vi "UHR-Fleezers Control (host) -Leonardo 04-2018 V2_sym.vi"(0 "Tab Control":T5(tab)=enum."Trap Control (RF)") -> ()   [LabVIEW 2013] (continued)
                      n1852 = Delete From Array(array=w3581, index=0) -> (array with subset deleted=w3579:cluster{"f0":dbl, "df":dbl, "magnitude":dbl[]}[])  [unwired: 1 in, 1 out]
                    }
                  }
                }
                frame True {
                  n1853 = Build Array(w3583) -> (w3582:cluster{"f0":dbl, "df":dbl, "magnitude":dbl[]}[])
                }
              }
              n1854 = for {
                tunnel: w3553 -> [w3572] mode=indexing
                tunnel: [w3571] -> w3563 mode=indexing
                workers-P: _ -> [_]
                n1855 = Unbundle By Name(w3572) -> ("magnitude"=w3571:dbl[])
              }
              n1856 = Transpose 2D Array(2D array=w3563) -> (transposed array=w3562:dbl[][])
              n1857 = for {
                tunnel: w3562 -> [w3570] mode=indexing
                tunnel: [w3569] -> w3561 mode=indexing
                workers-P: _ -> [_]
                n1858 = Add Array Elements(numeric array=w3570) -> (sum=w3569:dbl)
              }
              n1859 = Select(t=w3556, s=w3557, f=w3555) -> (s? t:f=w3554:dbl)
              n1860 = Divide(x=w3561, y=w3554) -> (x/y=w3559:dbl[])
              n1861 = Bundle By Name(cluster=w3560, "magnitude"=w3559) -> (w3558:cluster{"f0":dbl, "df":dbl, "magnitude":dbl[]})
            }
          }
        }
        n1862 = case shown="True" w3500 {
          tunnel: w3501 -> [w3532 w3538]
          tunnel: [w3532 w3533] -> w3499
          frame False {
          }
          frame True {
            n1863 = Array Subset(array=w3538, index (row)=0 ("index"), length (row)=4 ("length"), index (col)=0 ("index"), length (col)=1 ("length")) -> (w3533:T47)
          }
        }
        n1864 = feedback-in #9(w3499) -> ()
        n1865 = Split 1D Array(array=w3513, index=2) -> (first subarray=→"FFT 1":cluster{"f0":dbl, "df":dbl, "magnitude":dbl[]}[], second subarray=→"FFT 2":cluster{"f0":dbl, "df":dbl, "magnitude":dbl[]}[])
      }
    }
    n1866 = Index Array(array=w2395, index=1) -> (element=w2403:waveform(dbl))
    n1867 = case "For displaying the high resolution display (no downsampling)" shown="True" w2459 {
      tunnel: w2422 -> [_ w2741]
      frame False {
      }
      frame True {
        n1868 = Index Array(array=w2741, index="High Res. Display") -> (element=w2742:waveform(dbl))
        n1869 = call <vilib>:"Std Deviation and Variance.vi"("X"=w2742) -> ("mean"=w2749:dbl, "standard deviation"=w2754:dbl)  [unwired: 1 in, 1 out]
        "Mean Intensity" <- w2749
        "Sigma" <- w2754
        n1870 = Subtract(x=w2742, y=w2749) -> (x-y=w2748:waveform(dbl))
        n1871 = Select(t=w2748, s="Subtract mean", f=w2742) -> (s? t:f=→"1 Channel":waveform(dbl))
        n1872 = Divide(x=w2754, y=w2749) -> (x/y=→"Sigma/Mean":dbl)
        n1873 = feedback #10(1) -> (w2743:i32)
        n1874 = Greater Or Equal?(x=w2743, y="Slow mean N ave.") -> (x >= y?=w2756:bool)
        n1875 = Increment(x=w2743) -> (x+1=w2758:i32)
        n1876 = Select(t=1, s=w2756, f=w2758) -> (s? t:f=w2745:i32)
        n1877 = feedback-in #10(w2745) -> ()
        n1878 = feedback #11() -> (w2746:waveform(dbl))  [unwired: 1 out]
        n1879 = case shown="Default" w2743 {
          tunnel: [w2761 w2764] -> w2747
          tunnel: w2746 -> [w2763 _]
          tunnel: w2742 -> [w2762 w2764]
          frame Default {
            n1880 = call-poly <vilib>:"Append Waveforms.vi"("waveform B"=w2762, "waveform A"=w2763) -> ("waveform out"=w2761:waveform(dbl))  [unwired: 1 in, 8 out]
          }
          frame 1 {
          }
        }
        n1881 = feedback-in #11(w2747) -> ()
        n1882 = case shown="True" w2756 {
          tunnel: w2747 -> [_ w2760]
          frame False {
          }
          frame True {
            n1883 = call-poly <vilib>:"Mean.vi"("X"=w2760) -> ("mean"=→"Slow mean":dbl)  [unwired: 1 out]
          }
        }
      }
    }
    n1884 = case "For plotting results of scanning MCL" shown="True" w2529 {
      tunnel: w2528 -> [_ w2881]
      tunnel: w2452 -> [_ w2977]
      tunnel: w2537 -> [_ _]
      tunnel: w2422 -> [_ w2951]
      tunnel: w2397 -> [_ w2882]
      tunnel: w2396 -> [_ w2855]
      frame False {
      }
      frame True {
        w2862 = u32 0 items=["Horizontal", "Vertical", "Central", "1st Diagonal", "2nd Diagonal"] ("Type of Symmetry")
        w2890 = u32 0 items=["Horizontal", "Vertical", "Central", "1st Diagonal", "2nd Diagonal"] ("Type of Symmetry")
        w2893 = u32 0 items=["Horizontal", "Vertical", "Central", "1st Diagonal", "2nd Diagonal"] ("Type of Symmetry")
        w2922 = u32 0 items=["Horizontal", "Vertical", "Central", "1st Diagonal", "2nd Diagonal"] ("Type of Symmetry")
        n1885 = Index Array(array=w2951, index=10) -> (element=w2957:waveform(dbl))
        n1886 = Index Array(array=w2951, index=11) -> (element=w2954:waveform(dbl))
        n1887 = local read "Cycles/step (MCL)"() -> (w2907:u64)
        n1888 = Index Array(array=w2951, index="Channel") -> (element=w2953:waveform(dbl))
        n1889 = Unbundle(w2855) -> ("New Image"=w2854:T3, "New Image"=w2853:T3, "New Image"=w2852:T3, "New Image"=w2851:T3)
        n1890 = Unbundle By Name(w2957) -> ("Y"=w2909:dbl[])
        n1891 = Unbundle By Name(w2954) -> ("Y"=w2911:dbl[])
        n1892 = Unbundle By Name(w2953) -> ("Y"=w2916:dbl[])
        n1893 = call "downsample 1D array - double.vi"("Ave N"=w2907, "Array In"=w2909) -> ("Array Out"=w2908:dbl[])  [unwired: 1 out]
        n1894 = call "downsample 1D array - double.vi"("Ave N"=w2907, "Array In"=w2911) -> ("Array Out"=w2910:dbl[])  [unwired: 1 out]
        n1895 = call "downsample 1D array - double.vi"("Ave N"=w2907, "Array In"=w2916) -> ("Array Out"=w2915:dbl[])  [unwired: 1 out]
        n1896 = feedback #12(w2977) -> (w2978:dbl[])
        n1897 = Build Array (concatenate)(w2978, w2977) -> (w2959:dbl[])
        n1898 = feedback #13(w2882) -> (w2884:dbl[])
        n1899 = Build Array (concatenate)(w2884, w2882) -> (w2883:dbl[])
        n1900 = local read "Scan steps (MCL)"() -> (w2864:u64)
        n1901 = Select(t=w2977, s=w2881, f=w2959) -> (s? t:f=w2963:dbl[])
        n1902 = feedback-in #12(w2963) -> ()
        n1903 = Select(t=w2882, s=w2881, f=w2883) -> (s? t:f=w2865:dbl[])
        n1904 = feedback-in #13(w2865) -> ()
        n1905 = local read "Scan lines (y)"() -> (w2850:u64)
        n1906 = local read "N APD Samp/step"() -> (w2866:dbl)
        n1907 = feedback #14(w2908) -> (w2965:dbl[])
        n1908 = Build Array (concatenate)(w2965, w2908) -> (w2956:dbl[])
        n1909 = feedback #15(w2915) -> (w2975:dbl[])
        n1910 = Build Array (concatenate)(w2975, w2915) -> (w2974:dbl[])
        n1911 = feedback #16(w2910) -> (w2967:dbl[])
        n1912 = Build Array (concatenate)(w2967, w2910) -> (w2968:dbl[])
        n1913 = Select(t=w2908, s=w2881, f=w2956) -> (s? t:f=w2912:dbl[])
        n1914 = feedback-in #14(w2912) -> ()
        n1915 = Select(t=w2915, s=w2881, f=w2974) -> (s? t:f=w2914:dbl[])
        n1916 = feedback-in #15(w2914) -> ()
        n1917 = Select(t=w2910, s=w2881, f=w2968) -> (s? t:f=w2913:dbl[])
        n1918 = feedback-in #16(w2913) -> ()
        n1919 = Multiply(x=w2864, y=u64 2) -> (x*y=w2849:u64)
        n1920 = call "integrate 1D array interval - double.vi"("Ave N"=w2866, "Array In"=w2865) -> ("Array Out"=w2877:dbl[])  [unwired: 1 out]
        n1921 = call "integrate 1D array interval - double.vi"("Ave N"=w2866, "Array In"=w2963) -> ("Array Out"=w2962:dbl[])  [unwired: 1 out]
        n1922 = Array Size(array=w2877) -> (size(s)=w2878:i32)
        n1923 = Array Size(array=w2962) -> (size(s)=w2964:i32)
        n1924 = Multiply(x=w2850, y=w2849) -> (x*y=w2880:u64)
        n1925 = Multiply(x=w2850, y=w2849) -> (x*y=w2972:u64)
        n1926 = call-poly <vilib>:"Mean.vi"("X"=w2912) -> ("mean"=w2896:dbl)  [unwired: 1 out]
        n1927 = Subtract(x=w2880, y=w2878) -> (x-y=w2871:u64)
        n1928 = call-poly <vilib>:"Mean.vi"("X"=w2914) -> ("mean"=w2901:dbl)  [unwired: 1 out]
        n1929 = call-poly <vilib>:"Mean.vi"("X"=w2913) -> ("mean"=w2899:dbl)  [unwired: 1 out]
        n1930 = call-poly <vilib>:"Mean.vi"("X"=w2877) -> ("mean"=w2868:dbl)  [unwired: 1 out]
        n1931 = Subtract(x=w2972, y=w2964) -> (x-y=w2906:u64)
        n1932 = call-poly <vilib>:"Mean.vi"("X"=w2962) -> ("mean"=w2903:dbl)  [unwired: 1 out]
        n1933 = Initialize Array(1.0 ("element"), w2871) -> (w2867:dbl[])
        n1934 = Initialize Array(1.0 ("element"), w2906) -> (w2897:dbl[])
        n1935 = Multiply(x=w2867, y=w2868) -> (x*y=w2869:dbl[])
        n1936 = Multiply(x=w2897, y=w2899) -> (x*y=w2900:dbl[])
        n1937 = Multiply(x=w2897, y=w2901) -> (x*y=w2902:dbl[])
        n1938 = Multiply(x=w2897, y=w2896) -> (x*y=w2898:dbl[])
        n1939 = Multiply(x=w2897, y=w2903) -> (x*y=w2904:dbl[])
        n1940 = Build Array (concatenate)(w2912, w2898) -> (w2966:dbl[])
        n1941 = Build Array (concatenate)(w2914, w2902) -> (w2970:dbl[])
        n1942 = Build Array (concatenate)(w2913, w2900) -> (w2969:dbl[])
        n1943 = Build Array (concatenate)(w2877, w2869) -> (w2879:dbl[])
        n1944 = Build Array (concatenate)(w2962, w2904) -> (w2971:dbl[])
        n1945 = Reshape Array(w2966, w2850, w2849) -> (w2932:dbl[][])
        n1946 = Reshape Array(w2879, w2850, w2849) -> (w2875:dbl[][])
        n1947 = Reshape Array(w2970, w2850, w2849) -> (w2924:dbl[][])
        n1948 = Reshape Array(w2969, w2850, w2849) -> (w2939:dbl[][])
        n1949 = Reshape Array(w2971, w2850, w2849) -> (w2949:dbl[][])
        n1950 = Array Subset(array=w2939, index (col)=0 ("index"), length (col)=w2864) -> (w2944:dbl[][])  [unwired: 2 in]
        n1951 = Array Subset(array=w2939, index (col)=w2864) -> (w2942:dbl[][])  [unwired: 3 in]
        n1952 = Array Subset(array=w2924, index (col)=0 ("index"), length (col)=w2864) -> (w2930:dbl[][])  [unwired: 2 in]
        n1953 = Array Subset(array=w2924, index (col)=w2864) -> (w2928:dbl[][])  [unwired: 3 in]
        n1954 = Array Subset(array=w2875, index (col)=0 ("index"), length (col)=w2864) -> (w2874:dbl[][])  [unwired: 2 in]
        n1955 = Array Subset(array=w2875, index (col)=w2864) -> (w2872:dbl[][])  [unwired: 3 in]
        n1956 = Array Subset(array=w2949, index (col)=0 ("index"), length (col)=w2864) -> (w2948:dbl[][])  [unwired: 2 in]
        n1957 = Array Subset(array=w2949, index (col)=w2864) -> (w2946:dbl[][])  [unwired: 3 in]
        n1958 = Array Subset(array=w2932, index (col)=0 ("index"), length (col)=w2864) -> (w2937:dbl[][])  [unwired: 2 in]
        n1959 = Array Subset(array=w2932, index (col)=w2864) -> (w2935:dbl[][])  [unwired: 3 in]
        n1960 = for {
          tunnel: w2944 -> [w2986] mode=indexing
          tunnel: [w2985] -> w2943 mode=indexing
          workers-P: _ -> [_]
          n1961 = Reverse 1D Array(array=w2986) -> (reversed array=w2985:dbl[])
        }
        n1962 = for {
          tunnel: w2930 -> [w2982] mode=indexing
          tunnel: [w2981] -> w2929 mode=indexing
          workers-P: _ -> [_]
          n1963 = Reverse 1D Array(array=w2982) -> (reversed array=w2981:dbl[])
        }
        n1964 = for {
          tunnel: w2874 -> [w2980] mode=indexing
          tunnel: [w2979] -> w2873 mode=indexing
          workers-P: _ -> [_]
          n1965 = Reverse 1D Array(array=w2980) -> (reversed array=w2979:dbl[])
        }
        n1966 = for {
          tunnel: w2948 -> [w2988] mode=indexing
          tunnel: [w2987] -> w2947 mode=indexing
          workers-P: _ -> [_]
          n1967 = Reverse 1D Array(array=w2988) -> (reversed array=w2987:dbl[])
        }
        n1968 = for {
          tunnel: w2937 -> [w2984] mode=indexing
          tunnel: [w2983] -> w2936 mode=indexing
          workers-P: _ -> [_]
          n1969 = Reverse 1D Array(array=w2984) -> (reversed array=w2983:dbl[])
        }
        n1970 = Index Array(array=w2949, index (row)=0) -> (element=→"Waveform Graph":dbl[])  [unwired: 1 in]
        n1971 = Add(x=w2943, y=w2942) -> (x+y=w2941:dbl[][])
        n1972 = Add(x=w2929, y=w2928) -> (x+y=w2927:dbl[][])
        n1973 = Add(x=w2873, y=w2872) -> (x+y=w2857:dbl[][])
        n1974 = Add(x=w2947, y=w2946) -> (x+y=w2921:dbl[][])
        n1975 = Add(x=w2936, y=w2935) -> (x+y=w2934:dbl[][])
        n1976 = Divide(x=w2927, y=2) -> (x/y=w2925:dbl[][])
        n1977 = Divide(x=w2941, y=2) -> (x/y=w2886:dbl[][])
        n1978 = Divide(x=w2934, y=2) -> (x/y=w2888:dbl[][])
        n1979 = To Single Precision Float(number=w2921) -> (single precision float=w2920:sgl[][])
        n1980 = Transpose 2D Array(2D array=w2925) -> (transposed array=→"Data map":dbl[][])
        n1981 = To Single Precision Float(number=w2857) -> (single precision float=w2861:sgl[][])
        n1982 = To Single Precision Float(number=w2886) -> (single precision float=w2892:sgl[][])
        n1983 = To Single Precision Float(number=w2888) -> (single precision float=w2889:sgl[][])
        n1984 = call "IMAQ ArrayToImage"("Image Pixels (Float)"=w2920, "Image"=w2854) -> ("Image Out"=w2923:T3)  [unwired: 8 in, 1 out]
        n1985 = call "IMAQ ArrayToImage"("Image Pixels (Float)"=w2861, "Image"=w2853) -> ("Image Out"=w2863:T3)  [unwired: 8 in, 1 out]
        n1986 = call "IMAQ ArrayToImage"("Image Pixels (Float)"=w2892, "Image"=w2852) -> ("Image Out"=w2894:T3)  [unwired: 8 in, 1 out]
        n1987 = call "IMAQ ArrayToImage"("Image Pixels (Float)"=w2889, "Image"=w2851) -> ("Image Out"=w2891:T3)  [unwired: 8 in, 1 out]
        n1988 = call "IMAQ Symmetry"("Type of Symmetry"=w2922, "Image Src"=w2923) -> ("Image Dst Out"=w2918:T3)  [unwired: 3 in, 1 out]
        n1989 = call "IMAQ Symmetry"("Type of Symmetry"=w2862, "Image Src"=w2863) -> ("Image Dst Out"=w2859:T3)  [unwired: 3 in, 1 out]
        n1990 = call "IMAQ Symmetry"("Type of Symmetry"=w2893, "Image Src"=w2894) -> ("Image Dst Out"=→"Detection Laser X":T3)  [unwired: 3 in, 1 out]
        n1991 = call "IMAQ Symmetry"("Type of Symmetry"=w2890, "Image Src"=w2891) -> ("Image Dst Out"=→"Detection Laser Y":T3)  [unwired: 3 in, 1 out]
        n1992 = call "IMAQ Set Simple Calibration"("Calibration Axis Info"=T37 {"Origin Pixel"={"X"=0.0, "Y"=0.0}, "Angle Relative to Horizontal (deg)"=0.0, "Axis Reference"=0}, "Grid Descriptor"=T38 {"X Step"=0.3, "Y Step"=0.3, "Unit"=enum."Undefined"}, "Image"=w2918) -> ("Calibrated Image"=→"APD 1":T3)  [unwired: 7 in, 1 out]
        n1993 = call "IMAQ Set Simple Calibration"("Calibration Axis Info"=T37 {"Origin Pixel"={"X"=0.0, "Y"=0.0}, "Angle Relative to Horizontal (deg)"=0.0, "Axis Reference"=0}, "Grid Descriptor"=T38 {"X Step"=0.3, "Y Step"=0.3, "Unit"=enum."Undefined"}, "Image"=w2859) -> ("Calibrated Image"=→"APD 2":T3)  [unwired: 7 in, 1 out]
      }
    }
    n1994 = Subtract(x=w2403, y="APD 2 Offset") -> (x-y=w2400:waveform(dbl))
    n1995 = Subtract(x=w2405, y="APD 1 Offset") -> (x-y=w2401:waveform(dbl))
    n1996 = Index Array(array=w2420, index=3) -> (element=w2479:waveform(dbl))
    n1997 = Index Array(array=w2420, index=6) -> (element=w2476:waveform(dbl))
    n1998 = Build Array(w2401, w2400) -> (→"APD Chart":waveform(dbl)[])
    n1999 = Array Size(array=w2469) -> (size(s)=w2517:i32)
    n2000 = call <vilib>:"Std Deviation and Variance.vi"("X"=w2413) -> ("standard deviation"=w2412:dbl)  [unwired: 1 in, 2 out]
    n2001 = Add Array Elements(numeric array=w2413) -> (sum=w2415:u32)
    n2002 = Add Array Elements(numeric array=w2469) -> (sum=w2527:u32)
    n2003 = call <vilib>:"Std Deviation and Variance.vi"("X"=w2469) -> ("standard deviation"=w2468:dbl)  [unwired: 1 in, 2 out]
    n2004 = Divide(x=w2412, y=w2411) -> (x/y=w2408:dbl)
    "Rate sigma (Hz) 2" <- w2408
    n2005 = Multiply(x=w2411, y=w2517) -> (x*y=w2414:dbl)
    "Int. Time (s)" <- w2414
    n2006 = Divide(x=w2415, y=w2414) -> (x/y=w2409:dbl)
    "APD 2 Rate (Hz)" <- w2409
    n2007 = Divide(x=w2527, y=w2414) -> (x/y=w2466:dbl)
    "APD 1 Rate (Hz)" <- w2466
    n2008 = Divide(x=w2468, y=w2411) -> (x/y=w2467:dbl)
    "Rate sigma (Hz)" <- w2467
    n2009 = Divide(x=w2408, y=w2409) -> (x/y=→"Sigma/Mean 2":dbl)
    n2010 = Divide(x=w2467, y=w2466) -> (x/y=→"Sigma/Mean":dbl)
    n2011 = case shown="2" "Calibration" {
      tunnel: "T1 alpha_x (nm/V)" -> [_ w2817 w2838]
      tunnel: "T1 kappa_x (pN/nm)" -> [_ _ w2828]
      tunnel: "T2 alpha_x (nm/V)" -> [_ w2816 w2836]
      tunnel: "T2 kappa_x (pN/nm)" -> [_ _ w2829]
      tunnel: w2479 -> [w2799 w2814 w2834]
      tunnel: w2476 -> [w2798 w2812 w2832]
      tunnel: [w2799 w2811 w2831] -> w2269
      tunnel: [w2798 w2810 w2830] -> w2275
      tunnel: ["T1 X (V)" ("Label.Text") "T1 X (nm)" ("Label.Text") "T1 X (pN)" ("Label.Text")] -> w2497
      tunnel: ["T2 X (V)" ("Label.Text") "T2 X (nm)" ("Label.Text") "T2 X (pN)" ("Label.Text")] -> w2496
      tunnel: ["Position (V)" ("Label.Text") "Position (nm)" ("Label.Text") "Force (pN)" ("Label.Text")] -> w2498
      tunnel: w2478 -> [_ w2802 w2821]
      tunnel: w2480 -> [_ w2805 w2823]
      tunnel: ["Mean (V)" ("Label.Text") "Mean (nm)" ("Label.Text") "Mean (pN)" ("Label.Text")] -> w2493
      tunnel: ["Difference (V)" ("Label.Text") "Difference (nm)" ("Label.Text") "Difference (pN)" ("Label.Text")] -> w2428
      frame 0, Default {
      }
      frame 1 {
        # "position"
        n2012 = Unbundle By Name(w2814) -> ("Y"=w2818:dbl[])
        n2013 = Unbundle By Name(w2812) -> ("Y"=w2803:dbl[])
        n2014 = Subtract(x=w2818, y=w2805) -> (x-y=w2806:dbl[])
        n2015 = Subtract(x=w2803, y=w2802) -> (x-y=w2804:dbl[])
        n2016 = Multiply(x=w2804, y=w2816) -> (x*y=w2813:dbl[])
        n2017 = Multiply(x=w2817, y=w2806) -> (x*y=w2815:dbl[])
        n2018 = Bundle By Name(cluster=w2812, "Y"=w2813) -> (w2810:waveform(dbl))
        n2019 = Bundle By Name(cluster=w2814, "Y"=w2815) -> (w2811:waveform(dbl))
      }
      frame 2 {
        # "force"
        n2020 = Unbundle By Name(w2834) -> ("Y"=w2839:dbl[])
        n2021 = Unbundle By Name(w2832) -> ("Y"=w2837:dbl[])
        n2022 = Subtract(x=w2837, y=w2821) -> (x-y=w2822:dbl[])
        n2023 = Subtract(x=w2839, y=w2823) -> (x-y=w2824:dbl[])
        n2024 = Compound Arithmetic op=MULTIPLY(w2822, w2836, w2829) -> (w2833:dbl[])
        n2025 = Compound Arithmetic op=MULTIPLY(w2828, w2838, w2824) -> (w2835:dbl[])
        n2026 = Bundle By Name(cluster=w2832, "Y"=w2833) -> (w2830:waveform(dbl))
        n2027 = Bundle By Name(cluster=w2834, "Y"=w2835) -> (w2831:waveform(dbl))
      }
    }
    n2028 = feedback-in #17("Calibration") -> ()
    n2029 = feedback #17(u16 1 ("Calibration")) -> (w2500:u16)
    n2030 = local read "Trap 2 Bead Size (nm)"() -> (w2308:dbl)
    n2031 = local read "Trap 1 Bead Size (nm)"() -> (w2307:dbl)
    n2032 = local read "AOM X Cal (nm/MHz)"() -> (w2305:dbl)
    n2033 = local read "Trap Delta (MHz)"() -> (w2304:dbl)
    n2034 = Not Equal?(x=w2500, y="Calibration") -> (x != y?=w2457:bool)
    n2035 = Multiply(x=w2305, y=w2304) -> (x*y=w2309:dbl)
    n2036 = Unbundle By Name(w2269) -> ("Y"=w2274:dbl[])
    n2037 = Unbundle By Name(w2275) -> ("Y"=w2273:dbl[])
    n2038 = Add(x=w2308, y=w2307) -> (x+y=w2311:dbl)
    n2039 = case shown="False" "Negate trap 2 force" {
      tunnel: [-1.0 1.0] -> w2486
      frame False {
      }
      frame True {
      }
    }
    n2040 = Unbundle By Name(w2479) -> ("Y"=w2482:dbl[])
    n2041 = Unbundle By Name(w2476) -> ("Y"=w2485:dbl[])
    n2042 = Divide(x=w2311, y=2.0) -> (x/y=w2306:dbl)
    n2043 = Subtract(x=w2274, y=w2273) -> (x-y=w2271:dbl[])
    n2044 = Subtract(x=w2482, y=w2480) -> (x-y=w2483:dbl[])
    n2045 = Subtract(x=w2485, y=w2478) -> (x-y=w2484:dbl[])
    n2046 = Divide(x=w2271, y=2.0) -> (x/y=w2270:dbl[])
    n2047 = Multiply(x=w2484, y="T2 alpha_x (nm/V)") -> (x*y=w2475:dbl[])
    n2048 = Multiply(x="T1 alpha_x (nm/V)", y=w2483) -> (x*y=w2474:dbl[])
    n2049 = Multiply(x=w2275, y=w2486) -> (x*y=w2487:waveform(dbl))
    n2050 = Bundle By Name(cluster=w2269, "Y"=w2270) -> (w2268:waveform(dbl))
    n2051 = case shown="True" "Read Lateness and Rel Phase" {
      tunnel: w2281 -> [w2765 w2787]
      tunnel: w2320 -> [w2766 w2786]
      tunnel: [w2765 w2785] -> w2472
      tunnel: [w2766 w2784] -> w2471
      frame False {
      }
      frame True {
        n2052 = xnode "Read/Write Control"("FPGA VI Reference In"=w2787, "error in"=w2786) -> ("FPGA VI Reference Out"=w2785:T20, "error out"=w2784:errorcluster, "GI Relative phase"=→"GI relative phase":i16, "Relative phase"=→"Relative phase (AI1)":i16, "AI Late Counter"=→"Late Counter (AI1)":u8, "GI Late Counter"=→"GI Late Counter":u8, "MCL Late Counter"=→"MCL Late Counter":u8, "MCL Relative Phase"=→"Relative Phase (MCL)":i16, "APD Acq Relative Phase"=→"APD Acq Relative Phase":i16, "APD 1 Gate Relative Phase"=→"APD 1 Gate Relative Phase":i16, "APD 2 Gate Relative Phase"=→"APD 2 Gate Relative Phase":i16, "APD Acq Late Counter"=→"APD Acq Late Counter":u16, "APD 1 Gate Late Counter"=→"APD 1 Gate Late Counter":u8, "APD 2 Gate Late Counter"=→"APD 2 Gate Late Counter":u8, "Green FB Relative Phase"=→"Relative phase (Green FB)":i16, "GI Relative phase"=→"GI relative phase 2":i16, "GI Late Counter 2"=→"GI Late Counter 2":u16, "Trap Pos FIFO Timeout"=→"Trap Pos FIFO Timeout":u16, "Trap AI FIFO Timeout"=→"Trap AI FIFO Timeout":u16)
      }
    }
    n2053 = Subtract(x=w2475, y=w2474) -> (x-y=w2303:dbl[])
    n2054 = call-poly <vilib>:"Mean.vi"("X"=w2303) -> ("mean"=w2310:dbl)  [unwired: 1 out]
    n2055 = Add(x=w2309, y=w2310) -> (x+y=w2313:dbl)
    n2056 = Subtract(x=w2313, y=w2306) -> (x-y=→"Tether Extension (nm, calculated)":dbl)
    n2057 = Unbundle By Name(w2275) -> ("Y"=w2266:dbl[])
    n2058 = Unbundle By Name(w2269) -> ("Y"=w2267:dbl[])
    n2059 = Build Array(w2269, w2487, w2268) -> (→"Force":waveform(dbl)[])
    n2060 = Subtract(x=w2303, y="Offset (nm)") -> (x-y=w2447:dbl[])
    n2061 = call-poly <vilib>:"Mean.vi"("X"=w2266) -> ("mean"=w2264:dbl)  [unwired: 1 out]
    "T2 X" <- w2264
    n2062 = call-poly <vilib>:"Mean.vi"("X"=w2267) -> ("mean"=w2265:dbl)  [unwired: 1 out]
    "T1 X" <- w2265
    n2063 = Subtract(x=w2267, y=w2266) -> (x-y=w2449:dbl[])
    n2064 = Bundle By Name(cluster=w2479, "Y"=w2447) -> (w2419:waveform(dbl))
    "Bead Separation" <- w2419
    n2065 = Divide(x=w2449, y=2.0) -> (x/y=→"Vec Mean of T1 T2":dbl[])
    n2066 = case shown="True" w2457 {
      tunnel: w2498 -> [_ w2792]
      tunnel: w2497 -> [_ w2791]
      tunnel: w2496 -> [_ w2790]
      tunnel: w2493 -> [_ w2789]
      tunnel: w2428 -> [_ w2788]
      frame False {
      }
      frame True {
        n2067 = property on="Force" class="WFChart (strict)"("YScale.NameLbl.Text"=w2792) -> ()  [unwired: 2 in, 2 out]
        n2068 = property on="T2 X" class="DigNum (strict)"("Caption.Text"=w2790) -> ()  [unwired: 2 in, 2 out]
        n2069 = property on="T1 X" class="DigNum (strict)"("Caption.Text"=w2791) -> ()  [unwired: 2 in, 2 out]
        n2070 = property on="Mean" class="DigNum (strict)"("Caption.Text"=w2789) -> ()  [unwired: 2 in, 2 out]
        n2071 = property on="Difference" class="DigNum (strict)"("Caption.Text"=w2788) -> ()  [unwired: 2 in, 2 out]
      }
    }
    n2072 = local read "Tether"() -> (w2451:bool)
    n2073 = Subtract(x=w2265, y=w2264) -> (x-y=w2495:dbl)
    n2074 = Add(x=w2265, y=w2264) -> (x+y=→"Difference":dbl)
    n2075 = feedback #18(w2447) -> (w2446:dbl[])
    n2076 = Divide(x=w2495, y=2.0) -> (x/y=w2278:dbl)
    "Mean" <- w2278
    n2077 = case shown="True" w2451 {
      tunnel: w2278 -> [_ w2724]
      frame False {
      }
      frame True {
        n2078 = Greater?(x="Lost Tether Alarm Threshold (pN)", y=w2724) -> (0:w2722:bool)
        n2079 = case shown="True" w2722 {
          frame False {
          }
          frame True {
            n2080 = flat-sequence {
              frame #0 {
                # "stop only if saving"
                n2081 = local read "Saving..."() -> (w2737:bool)
                n2082 = And(x=w2737, y="TA Cancel Save?") -> (x .and. y?=w2736:bool)
                n2083 = local write "Stop Saving"(w2736) -> ()
              }
              frame #1 {
                n2084 = case shown="True" "TA Green Off?" {
                  frame False {
                  }
                  frame True {
                    w2740 = FALSE ("Fl. Triggered...")
                    n2085 = local write "Fl. Triggered..."(w2740) -> ()
                    n2086 = property on="Green Laser ON/Interlacing" class="Bool (strict)"("Val(Sgnl)"=w2740) -> ()  [unwired: 2 in, 2 out]
                  }
                }
              }
            }
            n2087 = local read "Time tether formed"() -> (w2731:timestamp)
            n2088 = Get Date/Time In Seconds() -> (seconds since 1Jan1904=w2732:timestamp)
            n2089 = Subtract(x=w2732, y=w2731) -> (x-y=w2730:dbl)
            n2090 = Number To Decimal String(number=w2730) -> (decimal integer string=w2727:string)  [unwired: 1 out]
            n2091 = local read "Messages"() -> (w2734:string)
            n2092 = call <vilib>:"Beep.vi"() -> ()  [unwired: 3 in, 9 out]
            n2093 = Concatenate Strings("Lost tether (" ("Message to add"), w2727, " s)." ("string")) -> (w2729:string)
            n2094 = local write "Tether"(FALSE ("Tether")) -> ()
            n2095 = call "Update messages.vi"("Message to add"=w2729, "Old message string"=w2734) -> ("New message string"=w2733:string)
            n2096 = local write "Messages"(w2733) -> ()
            n2097 = property on="Trap Pos. FB ON" class="Bool (strict)"("Val(Sgnl)"=FALSE ("Value (Signaling)")) -> ()  [unwired: 2 in, 2 out]
          }
        }
      }
    }
    n2098 = Build Array (concatenate)(w2447, w2446) -> (w2445:dbl[])
    n2099 = Split 1D Array(array=w2445, index=w2331) -> (first subarray=w2441:dbl[])  [unwired: 1 out]
    n2100 = feedback-in #18(w2441) -> ()
    n2101 = call-poly <vilib>:"Mean.vi"("X"=w2441) -> ("mean"=w2440:dbl)  [unwired: 1 out]
    "Bead Mean (nm)" <- w2440
    n2102 = Subtract(x=w2441, y=w2440) -> (x-y=w2439:dbl[])
    n2103 = Square(x=w2439) -> (x^2=w2438:dbl[])
    n2104 = case shown="True" "Semi Passive ON" {
      tunnel: "Semi Passive mode" -> [_ w2605]
      tunnel: "Jump Force (pN)" -> [_ w2604]
      tunnel: w2278 -> [_ w2603]
      frame False {
      }
      frame True {
        n2105 = case shown="\"Use Feedback\"" w2605 {
          tunnel: w2604 -> [_ w2608 w2624]
          tunnel: w2603 -> [_ w2607 w2623]
          frame "None" {
          }
          frame "Use Feedback" {
            n2106 = local read "Target Force (pN)"() -> (w2610:dbl)
            n2107 = Less?(x=w2608, y=w2610) -> (x < y?=w2609:bool)
            n2108 = case shown="True" w2609 {
              tunnel: w2608 -> [w2617 w2620]
              tunnel: w2607 -> [w2616 w2619]
              tunnel: [w2615 w2618] -> w2606
              frame False {
                n2109 = Less?(x=w2617, y=w2616) -> (x < y?=w2615:bool)
              }
              frame True {
                n2110 = Greater?(x=w2620, y=w2619) -> (0:w2618:bool)
              }
            }
            n2111 = case shown="True" w2606 {
              frame False {
                n2112 = local read "Trap Pos. FB ON"() -> (w2611:bool)
                n2113 = case shown="True" w2611 {
                  frame False {
                  }
                  frame True {
                    n2114 = property on="Trap Pos. FB ON" class="Bool (strict)"("Val(Sgnl)"=FALSE) -> ()  [unwired: 2 in, 2 out]
                  }
                }
              }
              frame True {
                n2115 = local read "Trap Pos. FB ON"() -> (w2613:bool)
                n2116 = case shown="False" w2613 {
                  frame False {
                    n2117 = property on="Trap Pos. FB ON" class="Bool (strict)"("Val(Sgnl)"=TRUE) -> ()  [unwired: 2 in, 2 out]
                  }
                  frame True {
                  }
                }
              }
            }
          }
          frame "Sharp Jump" {
            n2118 = local read "Target Force (pN)"() -> (w2626:dbl)
            n2119 = Greater?(x=w2624, y=w2626) -> (0:w2625:bool)
            n2120 = case shown="True" w2625 {
              tunnel: w2624 -> [w2641 w2645]
              tunnel: w2623 -> [w2642 w2644]
              tunnel: [w2640 w2643] -> w2622
              frame False {
                n2121 = Greater?(x=w2642, y=w2641) -> (0:w2640:bool)
              }
              frame True {
                n2122 = Less?(x=w2645, y=w2644) -> (x < y?=w2643:bool)
              }
            }
            n2123 = Subtract(x=w2624, y=w2626) -> (x-y=w2621:dbl)
            n2124 = case shown="True" w2622 {
              tunnel: w2621 -> [_ w2632]
              frame False {
              }
              frame True {
                n2125 = local read "T1 kappa_x (pN/nm)"() -> (w2637:dbl)
                n2126 = local read "T2 kappa_x (pN/nm)"() -> (w2638:dbl)
                n2127 = Reciprocal(x="DNA stiffness (pN / nm)") -> (1/x=w2634:dbl)
                n2128 = Reciprocal(x=w2637) -> (1/x=w2636:dbl)
                n2129 = Reciprocal(x=w2638) -> (1/x=w2635:dbl)
                n2130 = Compound Arithmetic op=ADD(w2636, w2635, w2634) -> (w2633:dbl)
                n2131 = local read "AOM X Cal (nm/MHz)"() -> (w2631:dbl)
                n2132 = Multiply(x=w2633, y=w2632) -> (x*y=w2630:dbl)
                n2133 = local read "Trap Delta (MHz)"() -> (w2628:dbl)
                n2134 = Divide(x=w2630, y=w2631) -> (x/y=w2629:dbl)
                n2135 = Subtract(x=w2628, y=w2629) -> (x-y=w2627:dbl)
                n2136 = property on="Trap Delta (MHz)" class="DigNum (strict)"("Val(Sgnl)"=w2627) -> ()  [unwired: 2 in, 2 out]
              }
            }
          }
        }
      }
    }
    n2137 = call-poly <vilib>:"Mean.vi"("X"=w2438) -> ("mean"=w2437:dbl)  [unwired: 1 out]
    n2138 = Square Root(x=w2437) -> (sqrt(x)=w2436:dbl)
    n2139 = Multiply(x=10.0, y=w2436) -> (x*y=→"RMS (Ang)":dbl)
    n2140 = xnode "Read/Write Control"("FPGA VI Reference In"=w2472, "error in"=w2471) -> ("FPGA VI Reference Out"=w2581:T20, "error out"=w2575:errorcluster, "AI2 Y Sum Set 1"=w2571:i16, "AI2 Y Sum Set 2"=w2570:i16, "AI1 X Set 1"=w2365:fxp<+/-,16,1>, "AI1 X Set 2"=w2364:fxp<+/-,16,1>, "Trap Pos FB Int Signal"=→"Trap Pos FB Int Signal":fxp<+/-,24,9>, "Trap Pos FB Int-Norm Signal"=→"Trap Pos FB Int-Norm Signal":fxp<+/-,16,1>, "Trap Pos FB Action"=w2358:i64, "Scanning"=→"AOD Scanning":bool, "Scan I"=→"AOD Scan I":u64, "Scanning MCL"=w2573:bool, "Scan I (MCL)"=→"MCL Scan I":u64, "Green FB Signals"=w2512:T48, "BD1 amplitude 1 out"=w2263:u16, "BD1 amplitude 2 out"=w2248:u16)  [unwired: 1 out]
    "MCL Scanning" <- w2573
    "Trap Pos FB Action" <- w2358
    n2141 = local read "AI2 (V)"() -> (w2572:cluster{"Set 1":dbl, "Set 2":dbl})
    n2142 = Bundle By Name(cluster=w2572, "Set 1"=w2571, "Set 2"=w2570) -> (w2568:cluster{"Set 1":dbl, "Set 2":dbl})
    n2143 = Divide(x=w2358, y=327.67) -> (x/y=→"Action (%)":dbl)
    n2144 = local read "Trap X (AI1)"() -> (w2378:T1)
    n2145 = Divide(x=w2568, y=3276.7) -> (x/y=w2567:cluster{"Set 1":dbl, "Set 2":dbl})
    n2146 = local write "AI2 (V)"(w2567) -> ()
    n2147 = Bundle(cluster=w2378, "Trap 1"=w2365, "Trap 2"=w2364) -> (→"Trap X (AI1)":T1)
    n2148 = Scale By Power Of 2(n=i16 12, x=ext 1.0) -> (x*2^n=w2259:ext)
    n2149 = Subtract(x=w2259, y=ext 1.0) -> (x-y=w2256:ext)
    n2150 = Divide(x=w2512, y=3276.7) -> (x/y=w2508:T49)
    n2151 = Multiply(x=w2263, y=ext 100.0) -> (x*y=w2257:ext)
    n2152 = Unbundle By Name(w2508) -> ("Green FB Ch 0"=w2511:dbl, "Green FB Ch 1"=w2510:dbl, "Green FB Ch 2"=w2509:dbl)
    n2153 = local read "All FB On/Off"() -> (w2247:bool)
    n2154 = Divide(x=w2257, y=w2256) -> (x/y=w2246:ext)
    "Trap 1 amplitude" <- w2246
    n2155 = Scale By Power Of 2(n=i16 12, x=ext 1.0) -> (x*2^n=w2252:ext)
    n2156 = Subtract(x=w2252, y=ext 1.0) -> (x-y=w2255:ext)
    n2157 = Multiply(x=w2248, y=ext 100.0) -> (x*y=w2254:ext)
    n2158 = Divide(x=w2511, y=w2509) -> (x/y=w2507:dbl)
    n2159 = Divide(x=w2510, y=w2509) -> (x/y=w2506:dbl)
    n2160 = flat-sequence "To save data" {
      tunnel: [w3621] -> w2592
      tunnel: [w3622] -> w2591
      tunnel: w2543 -> [w3615]
      tunnel: w2443 -> [w3619]
      tunnel: ["Save Calibration"] -> w2564
      tunnel: w2561 -> [w3618]
      tunnel: [w3611] -> w2560
      tunnel: [w3608] -> w2559
      tunnel: [w3605] -> w2558
      tunnel: w2542 -> [w3607]
      tunnel: w2455 -> [w3601]
      tunnel: [w3601] -> w2454
      tunnel: ["Start Saving"] -> w2421
      tunnel: [w3595] -> w2347
      tunnel: [w3594] -> w2346
      tunnel: w2592 -> [w3856]
      tunnel: w2591 -> [w3855]
      tunnel: w2348 -> [w3854]
      tunnel: w2564 -> [w3853]
      tunnel: w2560 -> [w3851]
      tunnel: w2559 -> [w3850]
      tunnel: w2558 -> [w3849]
      tunnel: w2430 -> [w3848]
      tunnel: w2464 -> [w3847]
      tunnel: w2454 -> [w3846]
      tunnel: w2421 -> [w3845]
      tunnel: w2419 -> [w3844]
      tunnel: w2395 -> [w3843]
      tunnel: w2347 -> [w3842]
      tunnel: w2346 -> [w3841]
      tunnel: w2345 -> [w3840]
      frame #0 {
        n2161 = Or(x="Save N Sets", y="Start Saving") -> (x .or. y?=w3602:bool)
        n2162 = To Double Precision Float(number=w3618) -> (double precision float=w3612:dbl)
        n2163 = Build Array(w3602, "Save Calibration", w3615, w3607) -> (w3617:bool[])
        n2164 = Compound Arithmetic op=OR("Save Calibration", w3615, w3602, w3607) -> (w3620:bool)
        n2165 = Boolean Array To Number(Boolean array=w3617) -> (number=w3614:u32)
        n2166 = feedback #19(FALSE ("Save APD Data\nwith Trap Data")) -> (w3596:bool)
        n2167 = feedback #20(refnum<k0> refnum) -> (w3623:refnum<file>)
        n2168 = feedback #21(refnum<k0> refnum) -> (w3598:refnum<file>)
        n2169 = feedback #22(FALSE ("Save APD Data\nwith Trap Data")) -> (w3606:bool)
        n2170 = feedback #23(refnum<k0> refnum) -> (w3609:refnum<file>)
        n2171 = feedback #24(0) -> (w3625:i32)
        n2172 = feedback #25() -> (w3613:u32)  [unwired: 1 out]
        n2173 = case shown="True" w3620 {
          tunnel: [w3632 1] -> w3621
          tunnel: w3625 -> [w3634 _]
          tunnel: [w3633 w3652] -> w3622
          tunnel: w3623 -> [w3633 _]
          tunnel: w3619 -> [_ w3672]
          tunnel: w3612 -> [_ w3670]
          tunnel: w3614 -> [_ w3673]
          tunnel: [w3631 w3651] -> w3611
          tunnel: w3613 -> [w3631 _]
          tunnel: [w3630 w3649] -> w3608
          tunnel: w3609 -> [w3630 _]
          tunnel: [w3629 w3648] -> w3605
          tunnel: w3606 -> [w3629 _]
          tunnel: "Start Saving" -> [_ w3646]
          tunnel: w3601 -> [_ w3645]
          tunnel: [w3628 w3636] -> w3594
          tunnel: w3598 -> [w3628 _]
          tunnel: [w3627 w3635] -> w3595
          tunnel: w3596 -> [w3627 _]
          frame False {
            n2174 = Increment(x=w3634) -> (x+1=w3632:i32)
          }
          frame True {
            w3642 = FALSE ("Start Saving")
            w3647 = 9.0  # File Version
            w3655 = FALSE ("prepend array or string size? (T)")
            w3653 = T30."big-endian, network order" ("byte order (0:big-endian, network order)")
            # "write file headers"
            n2175 = local read "BD 1 Frequency 1 (MHz)"() -> (w3669:dbl)
            n2176 = local read "BD 2 Frequency 1 (MHz)"() -> (w3668:dbl)
            n2177 = local read "BD 1 Frequency 2 (MHz)"() -> (w3667:dbl)
            n2178 = local read "BD 2 Frequency 2 (MHz)"() -> (w3666:dbl)
            n2179 = local read "BD 1 Frequency 3 (MHz)"() -> (w3665:dbl)
            n2180 = local read "BD 2 Frequency 3 (MHz)"() -> (w3664:dbl)
            n2181 = Array Size(array=w3645) -> (size(s)=w3644:i32)
            n2182 = To Double Precision Float(number=w3644) -> (double precision float=w3643:dbl)
            n2183 = local write "Save Calibration"(w3642) -> ()
            n2184 = local write "Start Saving"(w3642) -> ()
            n2185 = Build Array("Save APD Data\nwith Trap Data", "Save Trap Pos. Data") -> (w3639:bool[])
            n2186 = Boolean Array To Number(Boolean array=w3639) -> (number=w3638:u32)
            n2187 = Build Array(w3669, w3668, w3667, w3666, w3665, w3664) -> (w3663:dbl[])
            n2188 = case shown="8" w3673 {
              tunnel: w3672 -> [w3744 w3764 w3780 w3818]
              tunnel: w3643 -> [w3749 w3771 w3800 w3837]
              tunnel: w3670 -> [w3748 w3770 w3799 w3836]
              tunnel: [w3745 w3766 w3791 w3828] -> w3661
              tunnel: [w3736 "Cal sets to save" w3781 w3819] -> w3651
              tunnel: w3663 -> [w3746 w3767 w3793 w3830]
              tunnel: "Save APD Data\nwith Trap Data" -> [w3743 _ w3777 w3816]
              tunnel: [w3743 w3758 w3777 w3816] -> w3648
              tunnel: w3647 -> [w3739 w3759 w3775 w3814]
              tunnel: w3646 -> [w3738 _ _ _]
              tunnel: [w3729 w3758 w3774 w3804] -> w3635
              tunnel: "Save Trap Pos. Data" -> [w3729 _ w3774 w3804]
              tunnel: w3638 -> [w3728 _ w3773 w3803]
              frame 1, Default {
                # "timeseries"
                n2189 = case shown="True" "Profile" {
                  tunnel: [w3752 w3755] -> w3733
                  tunnel: [w3752 w3754] -> w3732
                  tunnel: [w3752 w3753] -> w3731
                  tunnel: [w3752 w3757] -> w3730
                  frame False {
                    w3752 = 0.0 ("f")
                  }
                  frame True {
                    n2190 = local read "Current Position"() -> (w3756:dbl[])
                    n2191 = local read "Y change (mm)"() -> (w3757:dbl)
                    n2192 = call "subVI_explode3array.vi"("Array"=w3756) -> ("x"=w3755:dbl, "y"=w3754:dbl, "z"=w3753:dbl)  [unwired: 12 in]
                  }
                }
                n2193 = local read "Save ave N"() -> (w3751:dbl)
                n2194 = Multiply(x=w3751, y=w3744) -> (x*y=w3750:dbl)
                n2195 = To Double Precision Float(number=w3728) -> (double precision float=w3742:dbl)
                n2196 = Build Array(w3739, w3744, w3750, w3749, w3748, 0.0 ("f")) -> (w3747:dbl[])
                n2197 = Build Array(w3742, w3733, w3732, w3731, w3730) -> (w3740:dbl[])
                n2198 = Select(t=u32 4000000000, s=w3738, f="N sets to save") -> (s? t:f=w3736:u32)
                n2199 = Build Array (concatenate)(w3747, w3746, w3740) -> (w3745:dbl[])
              }
              frame 2 {
                w3761 = 0.0 ("f")
                w3758 = FALSE ("Save APD Data\nwith Trap Data")
                # "calibration"
                n2200 = Boolean To (0,1)(Boolean=w3758) -> (0, 1=w3763:i16)
                n2201 = To Double Precision Float(number=w3763) -> (double precision float=w3762:dbl)
                n2202 = Build Array(w3762, w3761, w3761, w3761, w3761) -> (w3760:dbl[])
                n2203 = Build Array(w3759, w3764, w3764, w3771, w3770, 1.0 ("t")) -> (w3768:dbl[])
                n2204 = Build Array (concatenate)(w3768, w3767, w3760) -> (w3766:dbl[])
                "Calibrating Trap..." <- TRUE ("Calibrating...")
              }
              frame 4 {
                w3778 = 0.0 ("f")
                # "write file header for a trap \nraster scan"
                # "scan dir (x/y = 0/1)"
                # "cycles/step"
                # "n scans (f/b)"
                # "steps"
                # "freq. range"
                # "AOD raster scan"
                n2205 = local read "Number of F/B Scans (AOD)"() -> (w3785:u16)
                n2206 = local read "Cycles/step (AOD)"() -> (w3787:u64)
                n2207 = local read "Scan Range (MHz)"() -> (w3790:dbl)
                n2208 = local read "Scan steps (AOD)"() -> (w3789:u64)
                n2209 = local read "Scan BD"() -> (w3797:bool)
                n2210 = local read "Save ave N"() -> (w3802:dbl)
                n2211 = Boolean To (0,1)(Boolean=w3797) -> (0, 1=w3796:i16)
                n2212 = To Double Precision Float(number=w3785) -> (double precision float=w3784:dbl)
                n2213 = To Double Precision Float(number=w3789) -> (double precision float=w3788:dbl)
                n2214 = To Double Precision Float(number=w3787) -> (double precision float=w3786:dbl)
                n2215 = To Double Precision Float(number=w3796) -> (double precision float=w3795:dbl)
                n2216 = Multiply(x=w3802, y=w3780) -> (x*y=w3801:dbl)
                n2217 = To Double Precision Float(number=w3773) -> (double precision float=w3779:dbl)
                n2218 = Build Array(w3779, w3778, w3778, w3778, w3778) -> (w3776:dbl[])
                n2219 = local read "N sets should be saved"() -> (w3782:dbl)
                n2220 = Build Array(w3795, w3790, w3788, w3786, w3784) -> (w3792:dbl[])
                n2221 = Build Array(w3775, w3780, w3801, w3800, w3799, 2.0 ("t")) -> (w3794:dbl[])
                n2222 = Round Toward +Infinity(x=w3782) -> (ceil(x): smallest int >= x=w3783:dbl)
                n2223 = Build Array (concatenate)(w3794, w3793, w3776, w3792) -> (w3791:dbl[])
                n2224 = To Unsigned Long Integer(number=w3783) -> (unsigned 32bit integer=w3781:u32)
              }
              frame 8 {
                w3811 = 0.0 ("f")
                # "MCL raster scan"
                n2225 = local read "Number of scans (MCL)"() -> (w3806:u64)
                n2226 = local read "Scan lines (y)"() -> (w3805:u64)
                n2227 = local read "2D or 1D Scan"() -> (w3808:bool)
                n2228 = local read "Scan Range (V)\n(of steps)"() -> (w3827:dbl)
                n2229 = local read "Fast Scan Dir"() -> (w3834:bool)
                n2230 = local read "Cycles/step (MCL)"() -> (w3824:u64)
                n2231 = local read "Scan steps (MCL)"() -> (w3826:u64)
                n2232 = Select(t=w3805, s=w3808, f=w3806) -> (s? t:f=w3807:u64)
                n2233 = Boolean To (0,1)(Boolean=w3808) -> (0, 1=w3810:i16)
                n2234 = local read "Save ave N"() -> (w3839:dbl)
                n2235 = local read "Initial X"() -> (w3813:dbl)
                n2236 = local read "Initial Y"() -> (w3812:dbl)
                n2237 = To Double Precision Float(number=w3810) -> (double precision float=w3809:dbl)
                n2238 = Boolean To (0,1)(Boolean=w3834) -> (0, 1=w3833:i16)
                n2239 = To Double Precision Float(number=w3807) -> (double precision float=w3822:dbl)
                n2240 = To Double Precision Float(number=w3826) -> (double precision float=w3825:dbl)
                n2241 = To Double Precision Float(number=w3824) -> (double precision float=w3823:dbl)
                n2242 = To Double Precision Float(number=w3833) -> (double precision float=w3832:dbl)
                n2243 = Multiply(x=w3839, y=w3818) -> (x*y=w3838:dbl)
                n2244 = To Double Precision Float(number=w3803) -> (double precision float=w3817:dbl)
                n2245 = local read "N sets should be saved (MCL)"() -> (w3820:dbl)
                n2246 = Build Array(w3817, w3809, w3811, w3811, w3811) -> (w3815:dbl[])
                n2247 = Build Array(w3832, w3827, w3825, w3823, w3822, w3813, w3812) -> (w3829:dbl[])
                n2248 = Build Array(w3814, w3818, w3838, w3837, w3836, 3.0 ("t")) -> (w3831:dbl[])
                n2249 = Round Toward +Infinity(x=w3820) -> (ceil(x): smallest int >= x=w3821:dbl)
                n2250 = Build Array (concatenate)(w3831, w3830, w3815, w3829) -> (w3828:dbl[])
                n2251 = To Unsigned Long Integer(number=w3821) -> (unsigned 32bit integer=w3819:u32)
              }
            }
            n2252 = local read "Index"() -> (w3678:dbl)
            n2253 = call "Create new save file.vi"("Insert"="", "Ext"=".dat", "Index In"=w3678) -> ("Path Out"=w3637:path, "Index Out"=w3650:dbl)
            n2254 = local write "Save file name"(w3637) -> ()
            n2255 = local write "Index"(w3650) -> ()
            n2256 = local write "Save index"(w3650) -> ()
            n2257 = Array Size(array=w3661) -> (size(s)=w3662:i32)
            n2258 = Open/Create/Replace File(file path (use dialog)=w3637, operation (0:open)=T24."create", access (0:read/write)=enum16{"read/write", "read-only", "write-only"}."write-only") -> (refnum out=w3675:refnum<file>)  [unwired: 1 in, 4 out]
            n2259 = local write "Saving..."(TRUE ("Saving...")) -> ()
            n2260 = To Double Precision Float(number=w3662) -> (double precision float=w3660:dbl)
            n2261 = String Length(string="Comment (data description)") -> (length=w3658:i32)
            n2262 = To Double Precision Float(number=w3658) -> (double precision float=w3657:dbl)
            n2263 = Deny Access(7:w3675) -> (3:w3674:refnum<file>)  [unwired: 1 in, 2 out]
            n2264 = Build Array (concatenate)(w3660, w3661, w3657) -> (w3659:dbl[])
            n2265 = case "If fluorescence data to be saved" shown="True" w3648 {
              tunnel: w3637 -> [_ w3727]
              tunnel: [refnum<k0> refnum w3707] -> w3649
              frame False {
              }
              frame True {
                w3706 = 0.0
                n2266 = local read "APD Integration Time (s)"() -> (w3712:dbl)
                n2267 = local read "N APD Samp/step"() -> (w3705:dbl)
                n2268 = Path To String(path=w3727) -> (string=w3726:string)
                n2269 = String Length(string=w3726) -> (length=w3725:i32)
                n2270 = Subtract(x=w3725, y=4) -> (x-y=w3723:i32)
                n2271 = String Subset(string=w3726, length (rest)=w3723) -> (substring=w3722:string)  [unwired: 1 out]
                n2272 = Build Array(w3712, w3705, w3706, w3706, w3706, w3706, w3706, w3706) -> (w3709:dbl[])
                n2273 = Concatenate Strings(w3722, "_fl.dat" ("string")) -> (w3720:string)
                n2274 = Array Size(array=w3709) -> (size(s)=w3711:i32)
                n2275 = String To Path(string=w3720) -> (path=w3716:path)
                n2276 = Open/Create/Replace File(file path (use dialog)=w3716, operation (0:open)=T24."create", access (0:read/write)=enum16{"read/write", "read-only", "write-only"}."write-only") -> (refnum out=w3717:refnum<file>)  [unwired: 1 in, 4 out]
                n2277 = Deny Access(7:w3717) -> (3:w3713:refnum<file>)  [unwired: 1 in, 2 out]
                n2278 = To Double Precision Float(number=w3711) -> (double precision float=w3710:dbl)
                n2279 = Build Array (concatenate)(w3710, w3709) -> (w3708:dbl[])
                n2280 = Write to Binary File(file (use dialog)=w3713, data=w3708, 5:FALSE ("prepend array or string size? (T)"), 9:T30."big-endian, network order" ("byte order (0:big-endian, network order)")) -> (refnum out=w3707:refnum<file>)  [unwired: 1 in, 3 out]
              }
            }
            n2281 = case shown="True" w3635 {
              tunnel: w3637 -> [_ w3689]
              tunnel: [refnum<k0> refnum w3688] -> w3636
              frame False {
              }
              frame True {
                w3684 = 0.0 ("element")
                n2282 = Path To String(path=w3689) -> (string=w3703:string)
                n2283 = Build Array(w3684, w3684, w3684, w3684, w3684, w3684, w3684, w3684) -> (w3685:dbl[])
                n2284 = String Length(string=w3703) -> (length=w3702:i32)
                n2285 = Subtract(x=w3702, y=4) -> (x-y=w3700:i32)
                n2286 = Array Size(array=w3685) -> (size(s)=w3687:i32)
                n2287 = String Subset(string=w3703, length (rest)=w3700) -> (substring=w3699:string)  [unwired: 1 out]
                n2288 = To Double Precision Float(number=w3687) -> (double precision float=w3686:dbl)
                n2289 = Concatenate Strings(w3699, "_pos.dat" ("string")) -> (w3697:string)
                n2290 = Build Array (concatenate)(w3686, w3685) -> (w3683:dbl[])
                n2291 = String To Path(string=w3697) -> (path=w3693:path)
                n2292 = Open/Create/Replace File(file path (use dialog)=w3693, operation (0:open)=T24."create", access (0:read/write)=enum16{"read/write", "read-only", "write-only"}."write-only") -> (refnum out=w3694:refnum<file>)  [unwired: 1 in, 4 out]
                n2293 = Deny Access(7:w3694) -> (3:w3690:refnum<file>)  [unwired: 1 in, 2 out]
                n2294 = Write to Binary File(file (use dialog)=w3690, data=w3683, 5:FALSE ("prepend array or string size? (T)"), 9:T30."big-endian, network order" ("byte order (0:big-endian, network order)")) -> (refnum out=w3688:refnum<file>)  [unwired: 1 in, 3 out]
              }
            }
            n2295 = Write to Binary File(file (use dialog)=w3674, data=w3659, 5:w3655, 9:w3653) -> (refnum out=w3656:refnum<file>)  [unwired: 1 in, 3 out]
            n2296 = Write to Binary File(file (use dialog)=w3656, data="Comment (data description)", 5:w3655, 9:w3653) -> (refnum out=w3652:refnum<file>)  [unwired: 1 in, 3 out]
          }
        }
        n2297 = feedback-in #19(w3595) -> ()
        n2298 = feedback-in #20(w3622) -> ()
        n2299 = feedback-in #21(w3594) -> ()
        n2300 = feedback-in #22(w3605) -> ()
        n2301 = feedback-in #23(w3608) -> ()
        n2302 = feedback-in #24(w3621) -> ()
        n2303 = feedback-in #25(w3611) -> ()
      }
      frame #1 {
        n2304 = local read "Saving..."() -> (w3852:bool)
        n2305 = case shown="True" w3852 {
          tunnel: w3856 -> [_ w3866]
          tunnel: w3855 -> [_ w3880]
          tunnel: w3854 -> [_ w3876]
          tunnel: w3853 -> [_ w3875]
          tunnel: w3851 -> [_ w3874]
          tunnel: w3850 -> [_ w3869]
          tunnel: w3849 -> [_ w3868]
          tunnel: w3848 -> [_ w3867]
          tunnel: w3847 -> [_ w3865]
          tunnel: w3846 -> [_ w3863]
          tunnel: w3845 -> [_ w3862]
          tunnel: w3844 -> [_ w3861]
          tunnel: w3843 -> [_ w3860]
          tunnel: w3842 -> [_ w3859]
          tunnel: w3841 -> [_ w3858]
          tunnel: w3840 -> [_ w3857]
          frame False {
          }
          frame True {
            n2306 = Multiply(x=w3866, y=w3865) -> (x*y=→"Time (s)":dbl)
            n2307 = Less Or Equal?(x=w3866, y=w3874) -> (x <= y?=w3878:bool)
            n2308 = Or(x="Stop Saving", y="Abort save 2") -> (x .or. y?=w3870:bool)
            n2309 = Not(x=w3870) -> (.not. x?=w3879:bool)
            n2310 = And(x=w3878, y=w3879) -> (x .and. y?=w3877:bool)
            n2311 = case shown="True" w3877 {
              tunnel: w3880 -> [w3887 w3955]
              tunnel: [0.0 w3958] -> w3873
              tunnel: w3866 -> [_ w3956]
              tunnel: w3874 -> [_ w3957]
              tunnel: w3876 -> [_ w3952]
              tunnel: w3875 -> [_ _]
              tunnel: w3869 -> [w3885 w3945]
              tunnel: w3868 -> [w3884 w3946]
              tunnel: w3867 -> [_ w3944]
              tunnel: w3863 -> [_ w3943]
              tunnel: w3862 -> [_ w3897]
              tunnel: w3861 -> [_ w3936]
              tunnel: w3860 -> [_ w3914]
              tunnel: w3859 -> [w3882 w3895]
              tunnel: w3858 -> [w3883 w3894]
              tunnel: w3857 -> [_ w3891]
              frame False {
                w3881 = FALSE
                n2312 = Close File(refnum=w3887) -> ()  [unwired: 1 in, 2 out]
                n2313 = case shown="True" w3884 {
                  tunnel: w3885 -> [_ w3889]
                  frame False {
                  }
                  frame True {
                    n2314 = Close File(refnum=w3889) -> ()  [unwired: 1 in, 2 out]
                  }
                }
                n2315 = case shown="True" w3882 {
                  tunnel: w3883 -> [_ w3888]
                  frame False {
                  }
                  frame True {
                    n2316 = Close File(refnum=w3888) -> ()  [unwired: 1 in, 2 out]
                  }
                }
                n2317 = local write "Calibrating Trap..."(w3881) -> ()
                n2318 = call <vilib>:"Beep.vi"() -> ()  [unwired: 3 in, 9 out]
                n2319 = local write "Stop Saving"(w3881) -> ()
                n2320 = property on="Raster Scanning..." class="Bool (strict)"("Val(Sgnl)"=w3881) -> ()  [unwired: 2 in, 2 out]
                "Saving..." <- w3881
              }
              frame True {
                n2321 = local read "Calibrating Trap..."() -> (w3947:bool)
                n2322 = case "Write fl. data" shown="True" w3946 {
                  tunnel: w3945 -> [_ w3981]
                  tunnel: w3944 -> [_ w3980]
                  frame False {
                  }
                  frame True {
